vi "LWXPS_Open.vi"(7 "Device Key IN":string) -> (0 "LabVIEW error OUT":errorcluster, 1 "Returned error code":i32, 2 "Instrument Key OUT":string, 3 "XPS Reference OUT":refnum<k24>)   [LabVIEW 2020]
uses:
  C:/GEECS/Developers Version/builds/Device builds/XPS-RLD/Newport.XPS.CommandInterface.dll
  Newport.XPS.CommandInterface.dll
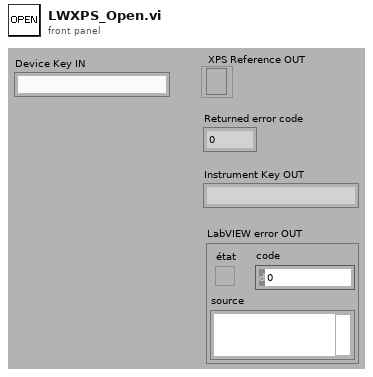
[diagram p1: front panel]
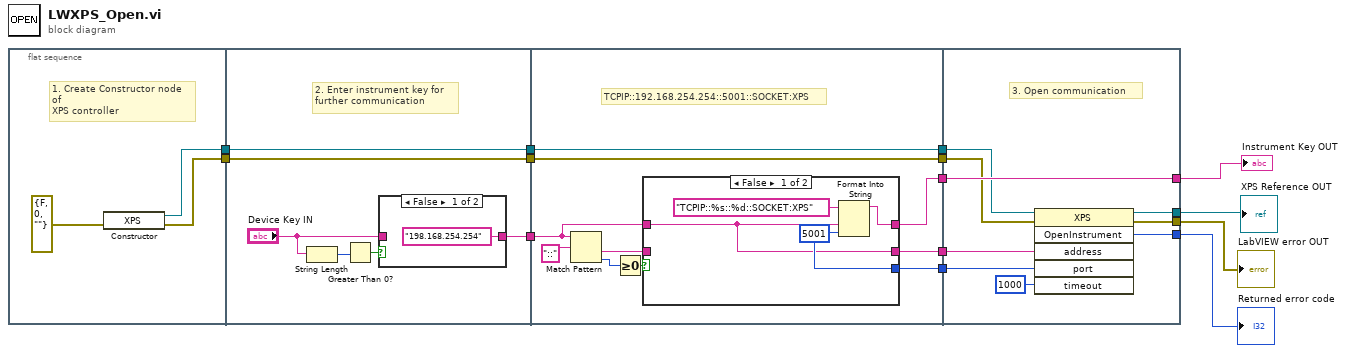
[diagram p0: block diagram]
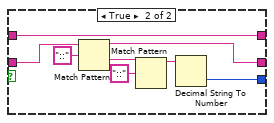
[diagram p3: hidden frame]
diagram:
  n1 = flat-sequence {
    tunnel: [w16] -> w11
    tunnel: [w15] -> w10
    tunnel: [w18] -> w14
    tunnel: [w20] -> w13
    tunnel: w11 -> [w20]
    tunnel: w10 -> [w18]
    tunnel: [w19] -> w12
    tunnel: w14 -> [w34]
    tunnel: w13 -> [w35]
    tunnel: w12 -> [w28]
    tunnel: [w27] -> w8
    tunnel: [w35] -> w7
    tunnel: [w34] -> w6
    tunnel: [w29] -> w5
    tunnel: [w26] -> w4
    tunnel: [w56] -> w9
    tunnel: w8 -> [w56]
    tunnel: w7 -> [w54]
    tunnel: w6 -> [w53]
    tunnel: w5 -> [w52]
    tunnel: w4 -> [w51]
    tunnel: [w50] -> w3
    tunnel: [w49] -> w2
    tunnel: [w48] -> w1
    frame #0 {
      # "1. Create Constructor node \nof \nXPS controller"
      n2 = constructor class="XPS"(error in=errorcluster {"status"=FALSE, "code"=0, "source"=""} ("entrée d'erreur (pas d'erreur)")) -> (reference out=w16:refnum<k24>, error out=w15:errorcluster)  [unwired: 2 in, 1 out]
    }
    frame #1 {
      # "2. Enter instrument key for \nfurther communication"
      n3 = String Length(string="Device Key IN") -> (length=w22:i32)
      n4 = Greater Than 0?(x=w22) -> (x > 0?=w23:bool)
      n5 = case shown="False" w23 {
        tunnel: ["198.168.254.254" ("Instrument Key IN") w25] -> w19
        tunnel: "Device Key IN" -> [_ w25]
        frame False {
        }
        frame True {
        }
      }
    }
    frame #2 {
      # "TCPIP::192.168.254.254::5001::SOCKET:XPS"
      n6 = Match Pattern(string=w28, regular expression="::" ("chaîne/car. recherché (-)")) -> (after substring=w33:string, offset past match=w30:i32)  [unwired: 1 in, 2 out]
      n7 = Greater Or Equal To 0?(x=w30) -> (x >= 0?=w31:bool)
      n8 = case shown="False" w31 {
        tunnel: w33 -> [_ w47]
        tunnel: [w36 w46] -> w29
        tunnel: [w37 w44] -> w27
        tunnel: w28 -> [w36 w44]
        tunnel: [w38 w40] -> w26
        frame False {
          w38 = 5001
          n9 = Format Into String(format string="TCPIP::%s::%d::SOCKET:XPS" ("chaîne de format"), w36, w38) -> (resulting string=w37:string)  [unwired: 2 in, 1 out]
        }
        frame True {
          n10 = Match Pattern(string=w47, regular expression="::" ("chaîne/car. recherché (-)")) -> (before substring=w46:string, after substring=w42:string)  [unwired: 1 in, 2 out]
          n11 = Match Pattern(string=w42, regular expression="::" ("chaîne/car. recherché (-)")) -> (before substring=w41:string)  [unwired: 1 in, 3 out]
          n12 = Decimal String To Number(string=w41) -> (number=w40:i32)  [unwired: 2 in, 1 out]
        }
      }
    }
    frame #3 {
      # "3. Open communication"
      n13 = invoke class="XPS" method="OpenInstrument"(reference=w54, error in=w53, "address"=w52, "port"=w51, "timeout"=1000) -> (reference out=w50:refnum<k24>, error out=w49:errorcluster, "OpenInstrument"=w48:i32)  [unwired: 1 in, 3 out]
    }
  }
  "LabVIEW error OUT" <- w2
  "Returned error code" <- w1
  "XPS Reference OUT" <- w3
  "Instrument Key OUT" <- w9
